vi "Particle_Main Function.vi"(6 "ForCalCalculaton In":T1, 7 "MAXParticle":i32, 8 "error in (no error)":errorcluster, 9 "Connectivity 4/8 (8)":bool=TRUE, 10 "Selected Particle":i32, 11 "Refnum in":T1) -> (0 "error out":errorcluster, 1 "Particle Reports (Real-World)":T2(array[cluster]) {"Orientation" format="%.2f"; "Dimensions"."Height" format="%.2f"; "Dimensions"."Width" format="%.2f"; "Center of Mass"."Y" format="%.2f"; "Center of Mass"."X" format="%.2f"; "Bounding Rect"."Bottom" format="%.2f"; "Bounding Rect"."Right" format="%.2f"; "Bounding Rect"."Top" format="%.2f"; "Bounding Rect"."Left" format="%.2f"; "Number of Holes" format="%.2f"; "Area" format="%.2f"}, 2 "Particle Report":T2(array[cluster]), 3 "Refnum out":T1, 4 "SearchSize":i32)   [LabVIEW 2019]
uses:
  <vilib>/vision/Image Controls.llb/IMAQ Image.ctl
  Controls/Parameter.ctl
  <vilib>/vision/NI_Vision_Development_Module.lvlib
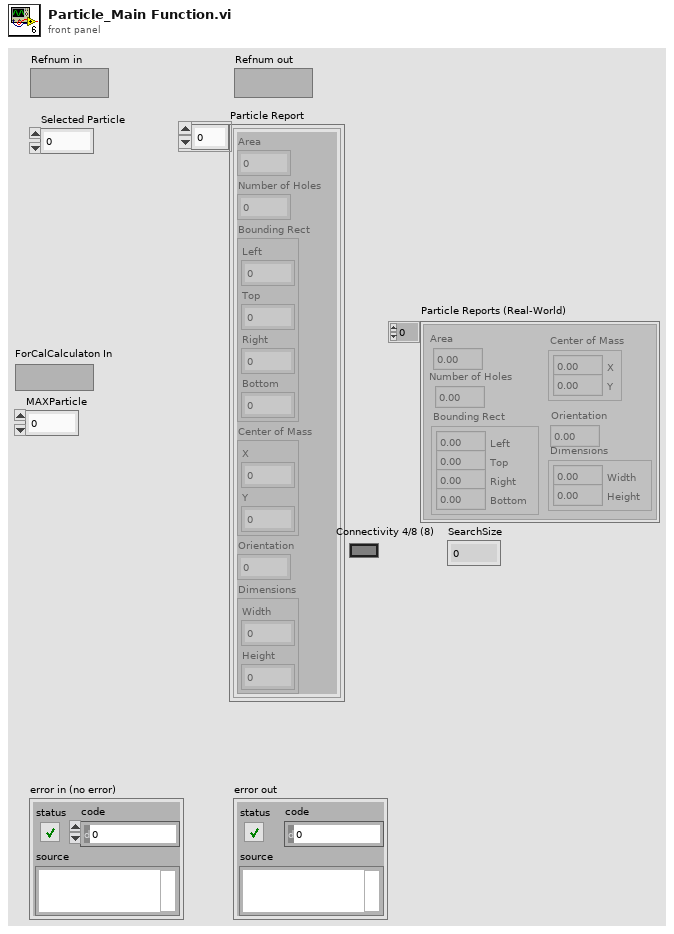
[diagram p1: front panel]
types:
  T1 = typedef "IMAQ Image.ctl" = refnum<image>
  T2 = cluster{"Area":dbl, "Number of Holes":dbl, "Bounding Rect":cluster{"Left":dbl, "Top":dbl, "Right":dbl, "Bottom":dbl}, "Center of Mass":cluster{"X":dbl, "Y":dbl}, "Orientation":dbl, "Dimensions":cluster{"Width":dbl, "Height":dbl}}[]
  T3 = cluster{"Area":dbl, "Number of Holes":dbl, "Bounding Rect":cluster{"Left":dbl, "Top":dbl, "Right":dbl, "Bottom":dbl}, "Center of Mass":cluster{"X":dbl, "Y":dbl}, "Orientation":dbl, "Dimensions":cluster{"Width":dbl, "Height":dbl}}
  T4 = typedef "Parameter.ctl" = enum16{"Initialize", "Write", "Read", "WriteAll", "Save", "Load"}
  T5 = typedef "ParameterData.ctl" = cluster{"Rotate Angle":dbl, "Rotate?":bool, "Calibration File Path":string, "Cal?":bool}
  T6 = cluster{"Left":dbl, "Top":dbl, "Right":dbl, "Bottom":dbl}
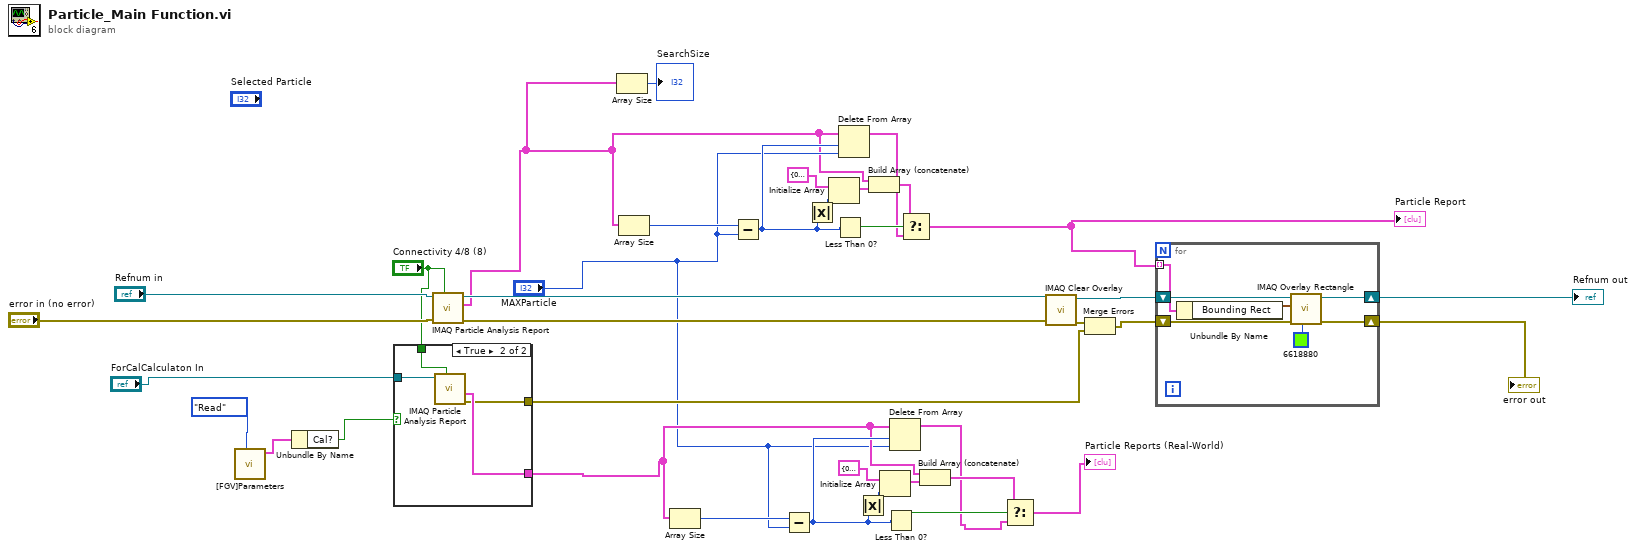
[diagram p0: block diagram]
diagram:
  n1 = call "[FGV]Parameters.vi"("Parameter"=Parameter."Read") -> ("ParameterData Out"=w24:T5)  [unwired: 9 in, 1 out]
  n2 = Unbundle By Name(w24) -> ("Cal?"=w23:bool)
  n3 = case shown="True" w23 {
    tunnel: "Connectivity 4/8 (8)" -> [_ w41]
    tunnel: "ForCalCalculaton In" -> [_ w40]
    tunnel: [_ w39] -> w6
    tunnel: [_ w38] -> w25
    frame False {
    }
    frame True {
      n4 = call "IMAQ Particle Analysis Report"("Connectivity 4/8 (8)"=w41, "Image"=w40) -> ("error out"=w38:errorcluster, "Particle Reports (Real-World)"=w39:T2)  [unwired: 4 in, 4 out]
    }
  }
  n5 = call "IMAQ Particle Analysis Report"("Connectivity 4/8 (8)"="Connectivity 4/8 (8)", "error in (no error)"="error in (no error)", "Image"="Refnum in") -> ("error out"=w32:errorcluster, "Particle Reports (Pixels)"=w2:T2, "Image Out (duplicate)"=w33:T1)  [unwired: 3 in, 3 out]
  n6 = Array Size(array=w2) -> (size(s)=→"SearchSize":i32)
  n7 = Array Size(array=w2) -> (size(s)=w22:i32)
  n8 = Array Size(array=w6) -> (size(s)=w7:i32)
  n9 = Subtract(x=w22, y="MAXParticle") -> (x-y=w19:i32)
  n10 = Subtract(x=w7, y="MAXParticle") -> (x-y=w9:i32)
  n11 = Absolute Value(x=w19) -> (abs(x)=w16:i32)
  n12 = Initialize Array(T3 {"Area"=0.0, "Number of Holes"=0.0, "Bounding Rect"={"Left"=0.0, "Top"=0.0, "Right"=0.0, "Bottom"=0.0}, "Center of Mass"={"X"=0.0, "Y"=0.0}, "Orientation"=0.0, "Dimensions"={"Width"=0.0, "Height"=0.0}} ("Particle Report"), w16) -> (w18:T2)
  n13 = Less Than 0?(x=w19) -> (x < 0?=w21:bool)
  n14 = Delete From Array(array=w2, length=w19, index="MAXParticle") -> (array with subset deleted=w20:T2)  [unwired: 1 out]
  n15 = Absolute Value(x=w9) -> (abs(x)=w12:i32)
  n16 = Build Array (concatenate)(w2, w18) -> (w17:T2)
  n17 = Initialize Array(T3 {"Area"=0.0, "Number of Holes"=0.0, "Bounding Rect"={"Left"=0.0, "Top"=0.0, "Right"=0.0, "Bottom"=0.0}, "Center of Mass"={"X"=0.0, "Y"=0.0}, "Orientation"=0.0, "Dimensions"={"Width"=0.0, "Height"=0.0}} ("Particle Report"), w12) -> (w10:T2)
  n18 = Less Than 0?(x=w9) -> (x < 0?=w8:bool)
  n19 = Delete From Array(array=w6, length=w9, index="MAXParticle") -> (array with subset deleted=w3:T2)  [unwired: 1 out]
  n20 = Select(t=w17, s=w21, f=w20) -> (s? t:f=w14:T2)
  "Particle Report" <- w14
  n21 = Build Array (concatenate)(w6, w10) -> (w11:T2)
  n22 = Select(t=w11, s=w8, f=w3) -> (s? t:f=→"Particle Reports (Real-World)":T2)
  n23 = call "IMAQ Clear Overlay"("error in (no error)"=w32, "Image"=w33) -> ("error out"=w37:errorcluster, "Image Out"=w36:T1)  [unwired: 8 in]
  n24 = Merge Errors(w37, w25) -> (w26:errorcluster)
  n25 = for {
    tunnel: w14 -> [w42] mode=indexing
    shift-right: [w44] -> w35
    shift-left: w26 -> [w48]
    shift-right: [w43] -> w34
    shift-left: w36 -> [w47]
    n26 = Unbundle By Name(w42) -> ("Bounding Rect"=w45:T6)
    n27 = call "IMAQ Overlay Rectangle"("Color"=u32 6618880, "error in (no error)"=w48, "Rectangle"=w45, "Image"=w47) -> ("error out"=w44:errorcluster, "Image Out"=w43:T1)  [unwired: 6 in]
  }
  "error out" <- w35
  "Refnum out" <- w34
